vi "Parse Command From Answer.vi"(8 "error in (no error)":errorcluster, 11 "JSON command":string) -> (0 "error out":errorcluster, 1 "Found?":bool, 3 "command string":string, 5 "returned answer":string)   [LabVIEW 2023, in "Communicator.lvclass"]
uses:
  Communicator.lvclass
  <vilib>/JDP Science/JSONtext/Next JSON Value.vi
  <vilib>/JDP Science/JSONtext/String Subset.vi
  <vilib>/JDP Science/JSONtext/Parsing/Advance past next JSON Value (inlined COPY).vi
  <vilib>/JDP Science/JSONtext/Parsing/Advance past whitespace.vi
  <vilib>/JDP Science/JSONtext/Parsing/Advance past String.vi
  <vilib>/JDP Science/JSONtext/Parsing/Advance past Number.vi
  <vilib>/JDP Science/JSONtext/Parsing/Advance past Line Ending.vi
  <vilib>/JDP Science/JSONtext/Parsing/Parse Full Path or Item Name.vi
  <vilib>/JDP Science/JSONtext/Parsing/Advance past Array.vi
  <vilib>/JDP Science/JSONtext/Parsing/Advance past Object.vi
  <vilib>/JDP Science/JSONtext/support/Error Cluster From Code.vi
  <vilib>/JDP Science/JSONtext/Offset/Find Item Locations by Path.vi
  <vilib>/JDP Science/JSONtext/JSONtext.lvlib
panel:
  # "Connector Pane"
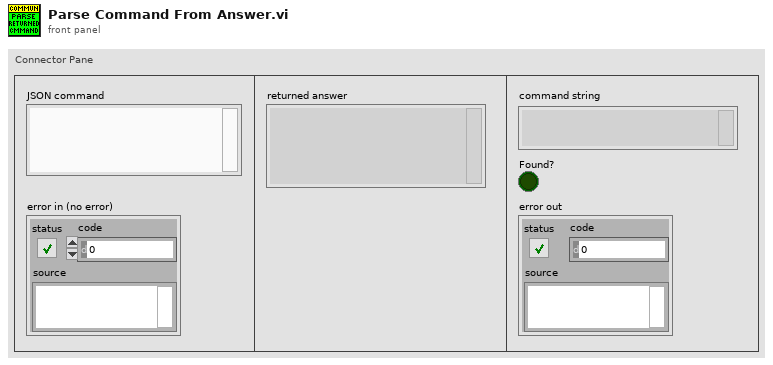
[diagram p1: front panel]
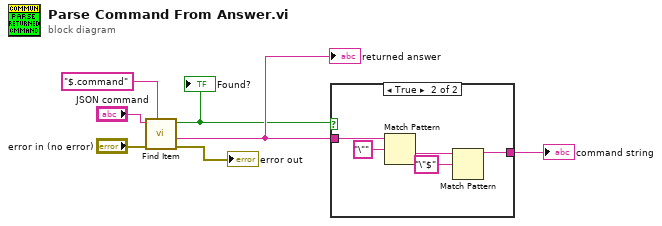
[diagram p0: block diagram]
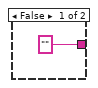
[diagram p2: hidden frame]
diagram:
  n1 = call <vilib>:"Find Item.vi"("$Path or Item Name"="$.command", "error in (no error)"="error in (no error)", "JSON"="JSON command") -> ("error out"=→"error out":errorcluster, "<JSON>"=w4:string, "Found"=w1:bool)  [unwired: 5 in, 1 out]
  "Found?" <- w1
  "returned answer" <- w4
  n2 = case shown="True" w1 {
    tunnel: ["" ("<JSON>") w9] -> w3
    tunnel: w4 -> [_ w12]
    frame False {
    }
    frame True {
      n3 = Match Pattern(string=w12, regular expression="\"" ("$Path or Item Name")) -> (after substring=w11:string)  [unwired: 1 in, 3 out]
      n4 = Match Pattern(string=w11, regular expression="\"$" ("$Path or Item Name")) -> (before substring=w9:string)  [unwired: 1 in, 3 out]
    }
  }
  "command string" <- w3
